vi "InitializeCore.vi"(8 "error in (no error)":errorcluster, 10 "Micron Args":T1, 11 "MicronServer in":refnum<class "ServiceBase.lvclass">) -> (0 "error out":errorcluster, 2 "MessageUserEvent":refnum<user-event>, 3 "MicronServer out":refnum<class "ServiceBase.lvclass">)   [LabVIEW 2019, in "MicronServer.lvlib" / "ServiceBase.lvclass"]
uses:
  ServiceBase.lvclass
  Message/MessageBase.lvclass
  Typedefs/MicronArgs.ctl
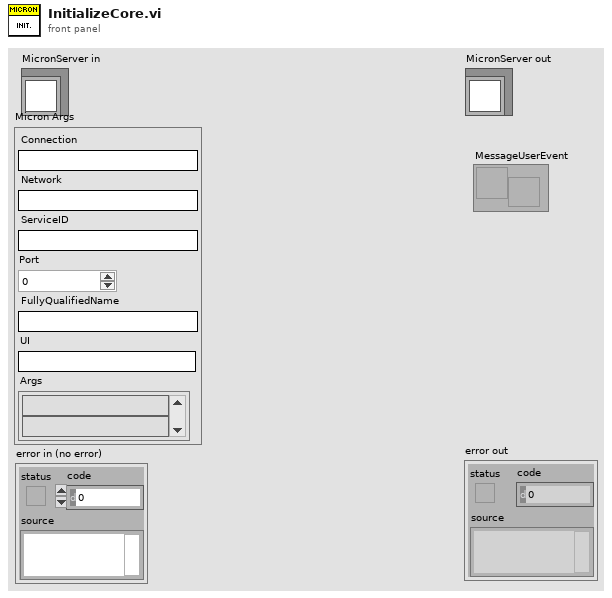
[diagram p1: front panel]
types:
  T1 = typedef "MicronServer.lvlib/ServiceBase.lvclass/MicronArgs.ctl" = cluster{"Connection":string, "Network":string, "ServiceID":string, "Port":i32, "FullyQualifiedName":string, "UI":string, "Args":string[]}
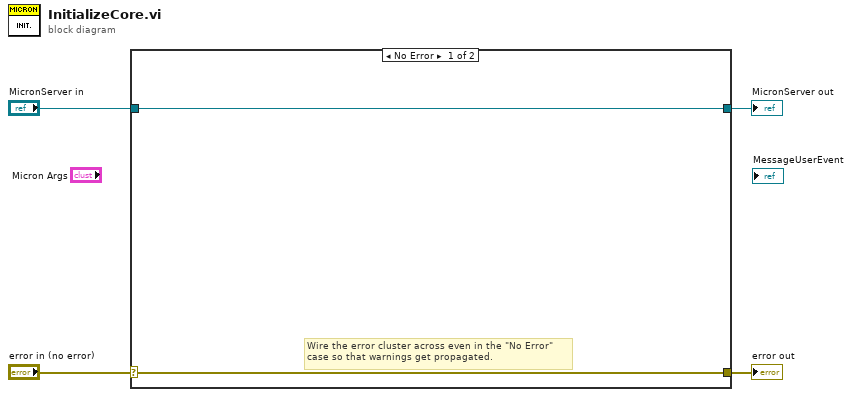
[diagram p0: block diagram]
diagram:
  n1 = case shown="No Error" "error in (no error)" {
    selector: "error in (no error)" -> [w5 w8]
    tunnel: [w5 w8] -> w3
    tunnel: [w6 w7] -> w1
    tunnel: "MicronServer in" -> [w6 w7]
    frame No Error {
      # "Wire the error cluster across even in the \"No Error\"\ncase so that warnings get propagated."
    }
    frame Error {
    }
  }
  "error out" <- w3
  "MicronServer out" <- w1
